vi "Network-Discovery Listener.vi"(0 "stop notifier":refnum<notifier>, 5 "discoveryPort":u16=10001, 7 "Discovery Events":T1) -> (15 "error out":errorcluster)   [LabVIEW 2020]
uses:
  Typedefs/Network-Discovery Events.ctl
  Typedefs/Network-Discovered Host.ctl
  Typedefs/Network-Server Beacon.ctl
  07eca581-5050-4c19-88ee-99fa771bf28b.vi
  Utility VIs/Controls/Utilities-Wait.vi/89bc9713-8f2c-40bd-a11f-1c800a437687.vi
  <vilib>/Utility/High Resolution Polling Wait.vi
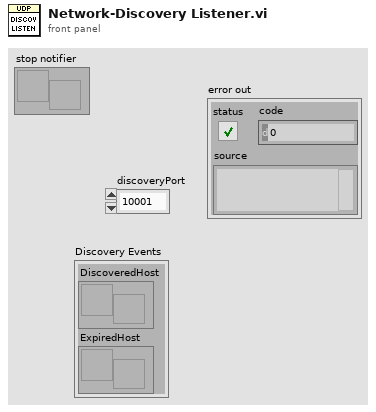
[diagram p1: front panel]
types:
  T1 = typedef "Network-Discovery Events.ctl" = cluster{"DiscoveredHost":refnum<user-event>, "ExpiredHost":refnum<user-event>}
  T2 = typedef "Network-Discovered Host.ctl" = cluster{"Beacon":T3, "Last Seen":timestamp}
  T3 = typedef "Network-Server Beacon.ctl" = cluster{"name":string, "addr":string, "port":u16, "ver":u16}
  T4 = cluster{"DiscoveryBeacon":T3, "seconds since 1Jan1904":timestamp}
  T5 = typedef "Network-Beacon Result.ctl" = enum16{"Ignored", "Updated", "Added"}
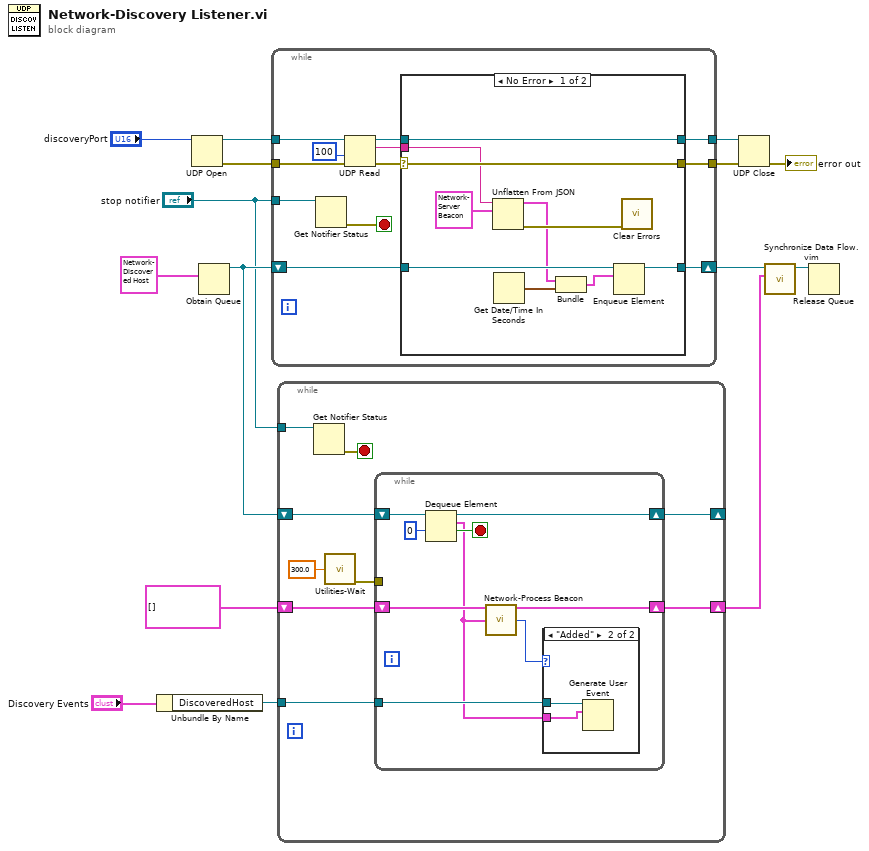
[diagram p0: block diagram]
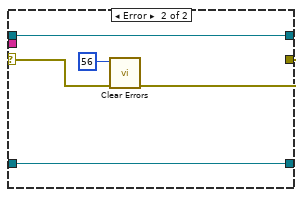
[diagram p3: hidden frame]
diagram:
  n1 = Unbundle By Name("Discovery Events") -> ("DiscoveredHost"=w5:refnum<user-event>)
  n2 = UDP Open(11:"discoveryPort") -> (port=w12:refnum<k16>, 0:w13:errorcluster)  [unwired: 4 in, 1 out]
  n3 = Obtain Queue(element data type=T2 {"Beacon"={"name"="", "addr"="", "port"=0, "ver"=10001}, "Last Seen"=timestamp(0 s since 1904-01-01)} ("DiscoveredHost")) -> (queue out=w9:refnum<queue>)  [unwired: 4 in, 2 out]
  n4 = while {
    tunnel: w12 -> [w27]
    tunnel: w13 -> [w26]
    tunnel: [w25] -> w14
    tunnel: [w24] -> w15
    tunnel: "stop notifier" -> [w19]
    shift-right: [w16] -> w4
    shift-left: w9 -> [w17]
    stop <- w18 stop-if-true
    n5 = Get Notifier Status(notifier=w19) -> (error out=w18:errorcluster)  [unwired: 1 in, 4 out]
    n6 = UDP Read(connection ID=w27, timeout ms (25000)=100, 8:w26) -> (data out=w21:string, error out=w22:errorcluster, 3:w20:refnum<k16>)  [unwired: 3 out]
    n7 = case shown="No Error" w22 {
      selector: w22 -> [w36 w42]
      tunnel: [w36 w40] -> w25
      tunnel: w21 -> [w35 _]
      tunnel: w20 -> [w37 w39]
      tunnel: [w37 w39] -> w24
      tunnel: w17 -> [w32 w38]
      tunnel: [w31 w38] -> w16
      frame No Error {
        n8 = Unflatten From JSON(JSON string=w35, type and defaults=T3 {"name"="", "addr"="192.168.1.98", "port"=57469, "ver"=10001} ("DiscoveryBeacon")) -> (value=w30:T3, error out=w33:errorcluster)  [unwired: 5 in]
        n9 = Get Date/Time In Seconds() -> (seconds since 1Jan1904=w29:timestamp)
        n10 = Bundle("DiscoveryBeacon"=w30, "seconds since 1Jan1904"=w29) -> (w28:T4)  [unwired: 1 in]
        n11 = Enqueue Element(queue=w32, element=w28) -> (queue out=w31:refnum<queue>)  [unwired: 2 in, 2 out]
        n12 = call <vilib>:"Clear Errors.vi"("error in (no error)"=w33) -> ()  [unwired: 5 in, 2 out]
      }
      frame Error {
        n13 = call <vilib>:"Clear Errors.vi"("error in (no error)"=w42, "specific error code to clear (0: all)"=56) -> ("error out"=w40:errorcluster)  [unwired: 4 in, 1 out]
      }
    }
  }
  n14 = while {
    shift-right: [w47] -> _
    shift-left: w9 -> [w49]
    shift-right: [w43] -> w2
    shift-left: T2[] [] ("Array") -> [w48]
    tunnel: w5 -> [w46]
    tunnel: "stop notifier" -> [w45]
    stop <- w44 stop-if-true
    n15 = Get Notifier Status(notifier=w45) -> (error out=w44:errorcluster)  [unwired: 1 in, 4 out]
    n16 = call "Utilities-Wait.vi"("milliseconds to wait"=300.0) -> ("error out"=w50:errorcluster)  [unwired: 14 in]
    n17 = while {
      tunnel: w50 -> [_]
      shift-right: [w58] -> w47
      shift-left: w49 -> [w60]
      shift-right: [w55] -> w43
      shift-left: w48 -> [w56]
      tunnel: w46 -> [w53]
      stop <- w57 stop-if-true
      n18 = Dequeue Element(queue=w60, timeout in ms (-1)=0) -> (queue out=w58:refnum<queue>, element=w52:T2, timed out?=w57:bool)  [unwired: 1 in, 1 out]
      n19 = call "Network-Process Beacon.vi"("Known Hosts in"=w56, "DiscoveredHost"=w52) -> ("Known Hosts out"=w55:T2[], "Beacon Result"=w54:T5)  [unwired: 12 in]
      n20 = case shown="\"Added\"" w54 {
        tunnel: w53 -> [_ w62]
        tunnel: w52 -> [_ w61]
        frame "Ignored", Default {
        }
        frame "Added" {
          n21 = Generate User Event(user event=w62, event data cluster=w61) -> ()  [unwired: 2 in, 2 out]
        }
      }
    }
  }
  n22 = UDP Close(connection ID=w15, 8:w14) -> (error out=→"error out":errorcluster)  [unwired: 1 out]
  n23 = call "Synchronize Data Flow.vim"("input 2"=w2, "input 1"=w4) -> ("output 1"=w3:refnum<queue>)  [unwired: 2 in, 3 out]
  n24 = Release Queue(queue=w3) -> ()  [unwired: 2 in, 3 out]
